vi "REPL_Comm.vi"(8 "REPL Name":string="Robot  REPL", 9 "CodeRef":refnum<vi>, 11 "Microprocessor in":T2) -> (3 "Microprocessor out":T2)   [LabVIEW 2016]
uses:
  uPythonX/uPythonX.xctl
  uPythonX/PythonData.ctl
  <vilib>/event_ctls.llb/eventvkey.ctl
  <vilib>/Utility/miscctls.llb/LVPointTypeDef.ctl
panel:
  in  "Find Port":bool
  out "return?":bool
  in  "Board":bool
  out "mouse down?":bool
  in  "Port":string
  in  "Delete":bool
  in  "New":bool
  in  "Files":u16(ring) items=["Current Code", "LPF2Class.py", "README.txt", "main.py"]
  in  "Ctrls":T1(ring)
  out "rows":string
  in  "View":u16(ring) items=["Complete Code"]
  in  "Spaces":bool
  in  "HelpCode":string
  in  "Stop Script":bool
  in  "Pause":bool
  in  "Help Button":bool
  in  "refresh":bool
  in  "Code":string
  out "Script":string
  in  "Copy":bool
  out "String":string
  in  "Run":bool
  out "FullCode":string
  in  "Clear":bool
  out "Origin":T3
  in  "Ctrl D":bool
  in  "Ctrl C":bool
  in  "Run DIrect":bool
  in  "Main":bool
  out "Console":string
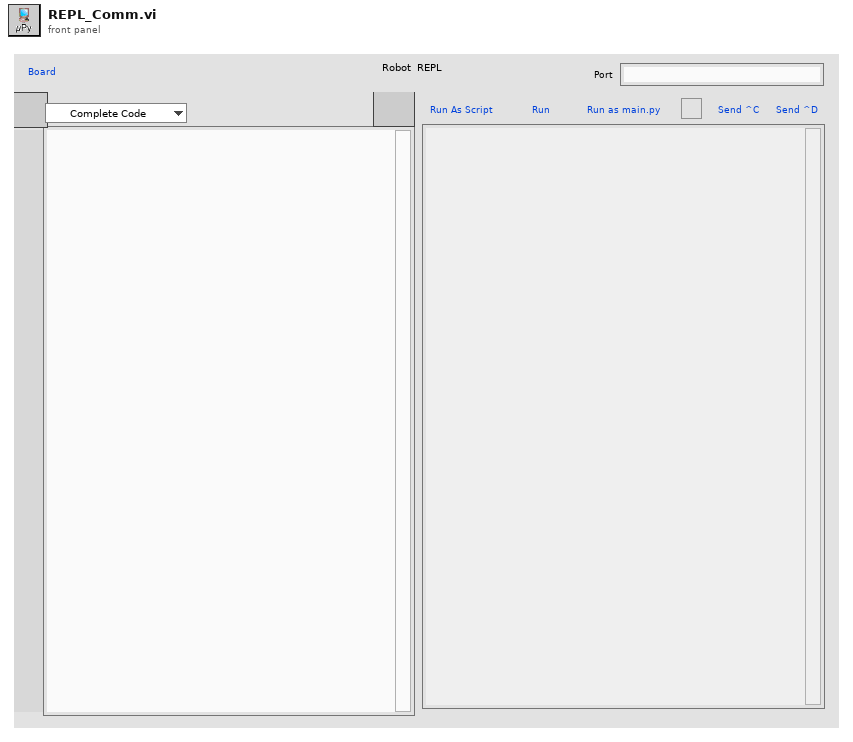
[diagram p1: front panel]
types:
  T1 = enum16{"File Control", "Save to PC", "Read from PC", "Save to MP as..."}
  T2 = cluster{"VISA Refnum in":refnum<visa-resource-name>, "Python Code":string}
  T3 = typedef "LVPointTypeDef.ctl" = cluster{"Horizontal":i16, "Vertical":i16}
  T4 = typedef "uPythonX.xctl/PythonData.ctl" = cluster{"Port":refnum<visa-resource-name>, "All Code":string}
  T5 = typedef "eventvkey.ctl" = enum16{"ASCII", "Enter", "Return", "Shift", "Ctrl", "Alt", "Cmd", "Opt", "Caps", "NumLock", "Clear", "Break", "Up", "Down", "Left", "Right", "Insert", "Delete", "Home", "End", "PageUp", "PageDown", "Escape", "Help", "Pause", "ScrollLock", "F1", "F2", "F3", "F4", "F5", "F6", "F7", "F8", "F9", "F10", "F11", "F12", "F13", "F14", "F15", "F16", "F17", "F18", "F19", "F20", "F21", "F22", "F23", "F24", "Play", "VolumeUp", "VolumeDown", "Mute", "Two Byte Char"}
  T6 = cluster{"Shift":bool, "Ctrl":bool, "Alt":bool, "Cmd":bool, "Opt":bool}
  T7 = cluster{"Char":i16, "VKey":T5, "ScanCode":i16, "Mods":cluster{"Num Pad":bool, "Menu Key":bool}, "PlatMods":cluster{"Shift":bool, "Ctrl":bool, "Alt":bool, "Cmd":bool, "Opt":bool}, "FocusObj":refnum<vi>}
  T8 = enum16{"Left Button", "Center Button", "Right Button", "Window Close"}
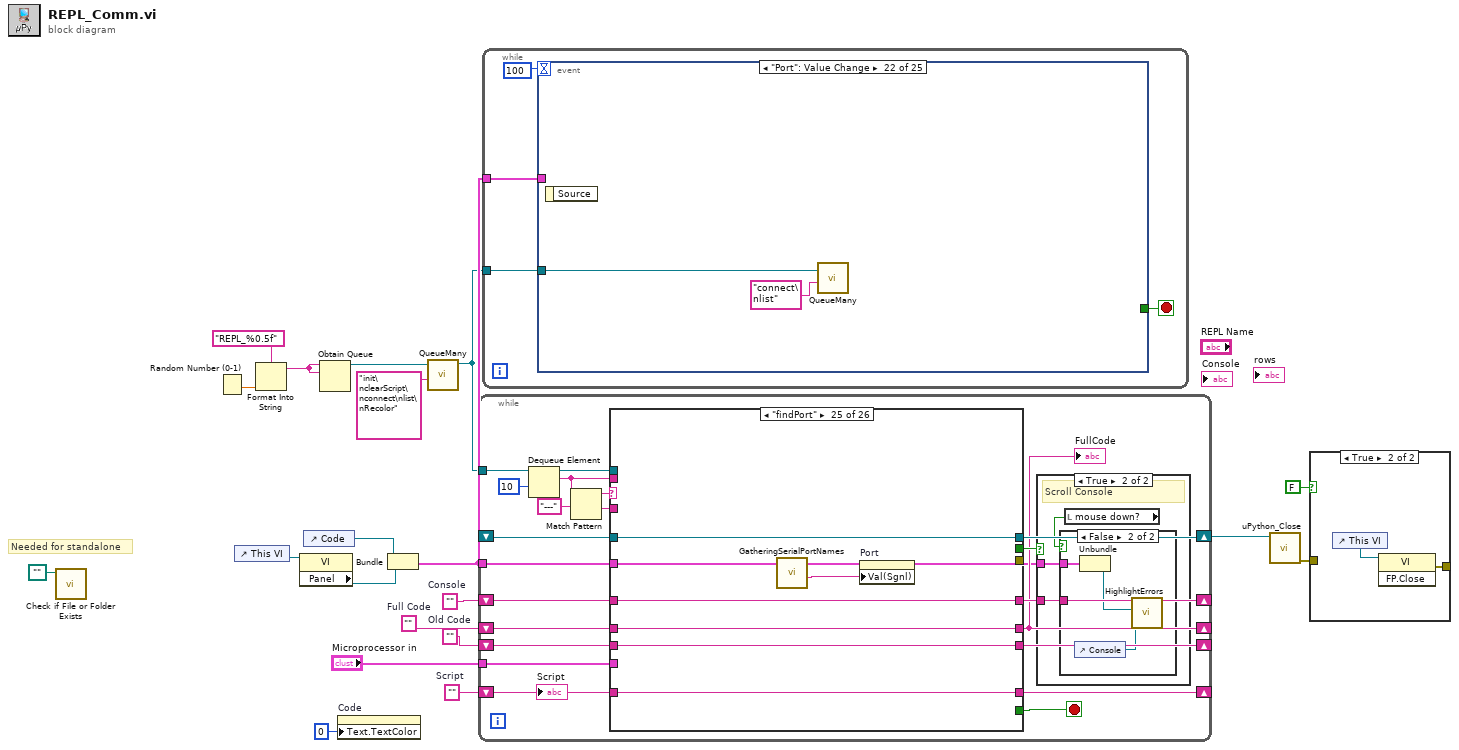
[diagram p0: block diagram]
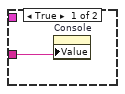
[diagram p4: hidden frame]
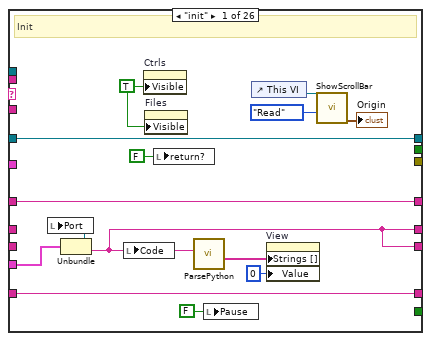
[diagram p5: hidden frame]
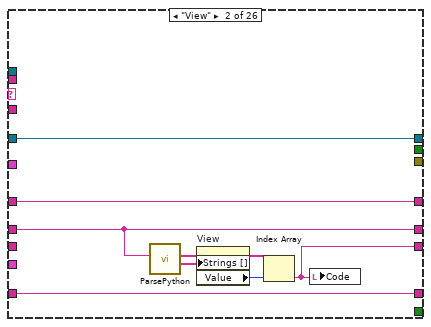
[diagram p6: hidden frame]
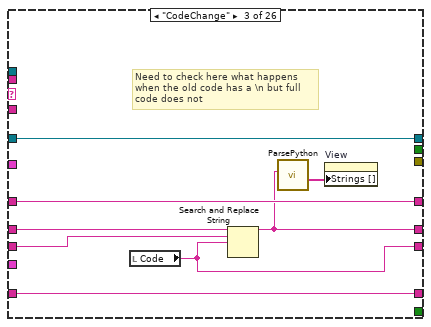
[diagram p7: hidden frame]
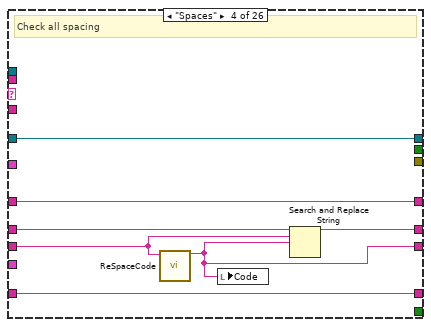
[diagram p8: hidden frame]
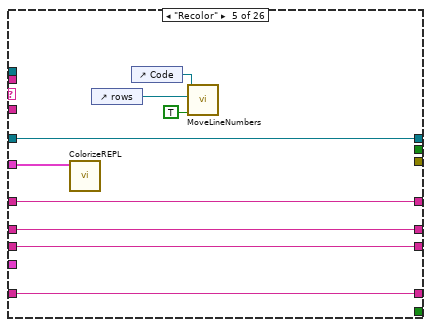
[diagram p9: hidden frame]
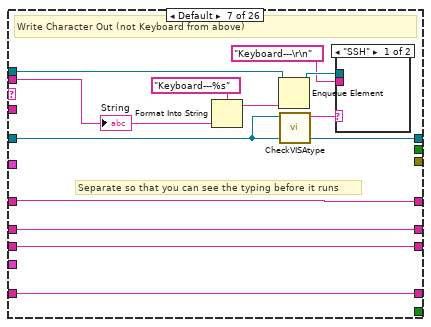
[diagram p11: hidden frame]
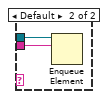
[diagram p12: hidden frame]
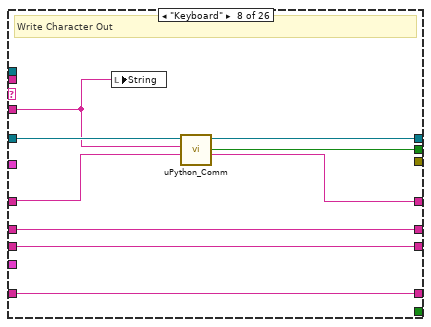
[diagram p13: hidden frame]
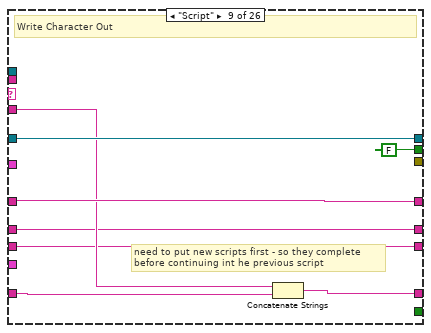
[diagram p14: hidden frame]
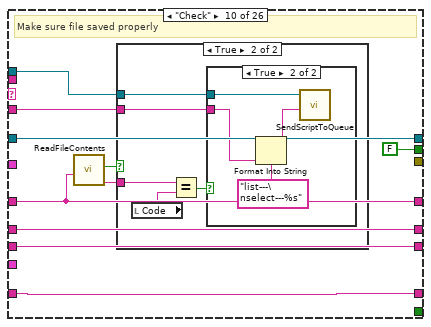
[diagram p15: hidden frame]
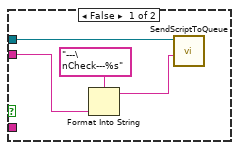
[diagram p16: hidden frame]
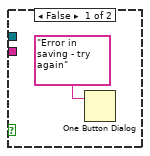
[diagram p17: hidden frame]
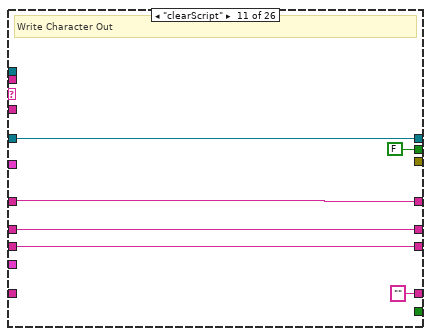
[diagram p18: hidden frame]
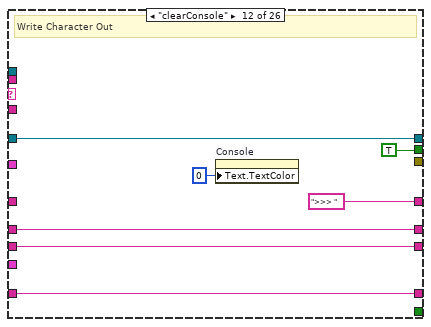
[diagram p19: hidden frame]
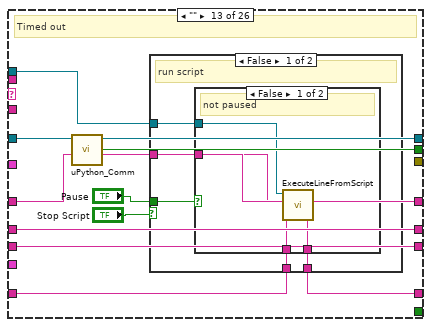
[diagram p20: hidden frame]
diagram:
  w6 = ""  # Old Code
  w7 = ""  # Full Code
  w15 = ""  # Script
  w16 = ""  # Console
  # "Needed for standalone"
  n1 = call <vilib>:"Check if File or Folder Exists.vi"("path"=path "") -> ()  [unwired: 8 in, 3 out]
  n2 = Random Number (0-1)() -> (number: 0 to 1=w10:dbl)
  n3 = control-ref of="This VI"() -> (w5:refnum<vi>)
  n4 = Format Into String(format string="REPL_%0.5f" ("name (unnamed)"), w10) -> (resulting string=w9:string)  [unwired: 2 in, 1 out]
  n5 = property class="VI"(reference=w5) -> ("Panel"=w3:refnum<vi>)  [unwired: 1 in, 2 out]
  n6 = control-ref of="Code"() -> (w4:refnum<vi>)
  n7 = Obtain Queue(name (unnamed)=w9, element data type=w9) -> (queue out=w19:refnum<queue>)  [unwired: 3 in, 2 out]
  n8 = property on="Code" class="Str"("Text.TextColor"=u32 0 ("Text.Text Colors:Text Color")) -> ()  [unwired: 2 in, 2 out]
  n9 = Bundle("Code"=w4, "Panel"=w3) -> (w20:cluster{"Code":refnum<vi>, "Panel":refnum<vi>})  [unwired: 1 in]
  n10 = call "QueueMany.vi"("Playlist"="init\nclearScript\nconnect\nlist\nRecolor" ("element"), "Queue in"=w19) -> ("Queue out"=w18:refnum<queue>)  [unwired: 9 in]
  n11 = while {
    tunnel: w18 -> [w41]
    shift-right: [w31] -> w17
    shift-left: _ -> [w39]
    shift-right: [w30] -> _
    shift-left: w16 -> [w32]
    shift-right: [w28] -> _
    shift-left: w15 -> [w27]
    tunnel: "Microprocessor in" -> [w26]
    shift-right: [w24] -> _
    shift-left: w7 -> [w25]
    shift-right: [w23] -> _
    shift-left: w6 -> [w22]
    tunnel: w20 -> [w21]
    stop <- w40 stop-if-true
    n12 = Dequeue Element(queue=w41, timeout in ms (-1)=10) -> (queue out=w37:refnum<queue>, element=w33:string)  [unwired: 1 in, 2 out]
    n13 = Match Pattern(string=w33, regular expression="---") -> (before substring=w35:string, after substring=w34:string)  [unwired: 1 in, 2 out]
    n14 = case shown="\"findPort\"" w35 {
      tunnel: [_ _ _ _ _ _ _ _ _ _ _ _ _ _ _ _ _ _ _ _ _ _ _ _ _ TRUE] -> w40
      tunnel: w39 -> [w63 w71 w79 w86 w95 w100 w102 w122 w131 w141 w161 w168 w178 _ w207 w221 w236 w244 w248 w276 w289 w300 w310 w316 w322 w336]
      tunnel: w37 -> [_ _ _ _ _ _ w105 _ _ w137 _ _ w169 _ w211 w218 w233 _ _ _ _ _ _ _ _ _]
      tunnel: w34 -> [_ _ _ _ _ _ _ w117 w126 w134 _ _ _ _ _ _ _ _ _ _ _ w301 _ _ _ _]
      tunnel: w33 -> [_ _ _ _ _ _ w107 _ _ _ _ _ _ _ _ _ _ _ _ _ _ _ _ _ _ _]
      tunnel: [w63 w71 w79 w86 w95 w100 w102 w120 w131 w141 w161 w168 w175 w203 w207 w221 w236 w244 w256 w280 w286 w300 w310 w316 w322 w336] -> w31
      tunnel: w32 -> [w62 w70 w78 w85 w94 w99 w111 w121 w130 w136 w160 _ w177 _ w210 w220 w235 w243 w251 w277 w290 w299 w312 w318 w324 w337]
      tunnel: [w62 w70 w78 w85 w94 w99 w111 w119 w130 w136 w160 ">>> " ("Console") w176 w201 w210 w220 w235 w243 w254 w264 w284 w299 w312 w318 w324 w337] -> w30
      tunnel: [_ _ _ _ _ _ _ _ _ _ _ _ _ w202 _ _ _ _ w253 w279 w285 _ _ _ _ _] -> _
      tunnel: [_ _ _ _ _ _ _ w118 FALSE ("Update?") FALSE ("Update?") FALSE ("Update?") TRUE ("Update?") w174 _ TRUE ("Update?") FALSE ("Update?") _ _ TRUE ("Update?") TRUE ("Update?") TRUE ("Update?") _ _ _ _ _] -> w29
      tunnel: [w61 w69 w77 w84 w92 w98 w112 w123 w128 w139 "" ("Script") w166 w180 w200 w212 w222 w237 w240 w262 w282 w292 w298 w311 w317 w323 w334] -> w28
      tunnel: w27 -> [w61 w69 w77 w84 w92 w98 w112 w123 w127 w139 _ w166 w179 w200 w212 w222 w237 w240 w262 w282 w292 w298 w311 w317 w323 w334]
      tunnel: w26 -> [w60 _ _ _ _ _ _ _ _ _ _ _ _ _ _ _ _ _ _ _ _ _ _ _ _ w333]
      tunnel: [w51 w67 w72 w80 w91 w97 w104 w116 w125 w133 w157 w164 w172 w198 w209 w217 w232 w242 w247 w275 w288 w294 w304 w314 w321 w328] -> w24
      tunnel: w25 -> [_ w67 w76 w83 w91 w97 w104 w116 w125 w133 w157 w164 w172 w198 w209 w217 _ w242 w247 w275 w288 w294 w304 w314 w321 w328]
      tunnel: [w51 w64 w74 w81 w93 w96 w103 w115 w124 w132 w156 w163 w171 w197 w208 w216 w232 w241 w246 w274 w287 w293 w303 w313 w320 w327] -> w23
      tunnel: w22 -> [_ _ w75 w82 w93 w96 w103 w115 w124 w132 w156 w163 w171 w197 w208 w216 _ w241 w246 w274 w287 w293 w303 w313 w320 w327]
      tunnel: w21 -> [_ _ _ _ w90 _ _ _ _ _ _ _ _ _ _ _ _ _ _ _ _ _ _ _ _ _]
      frame "init" {
        w58 = TRUE ("Visible")
        # "Init"
        n15 = Unbundle(w60) -> ("VISA Refnum in"=w54:refnum<visa-resource-name>, "Python Code"=w51:string)
        n16 = local write "Port"(w54) -> ()
        n17 = local write "Code"(w51) -> ()
        n18 = property on="Ctrls" class="Enum (strict)"("Visible"=w58) -> ()  [unwired: 2 in, 2 out]
        n19 = property on="Files" class="Ring (strict)"("Visible"=w58) -> ()  [unwired: 2 in, 2 out]
        n20 = local write "return?"(FALSE ("return?")) -> ()
        n21 = call "ParsePython.vi"("String"=w51) -> ("functions"=w53:string[])  [unwired: 8 in, 2 out]
        n22 = local write "Pause"(FALSE ("Pause")) -> ()
        n23 = control-ref of="This VI"() -> (w57:refnum<vi>)
        n24 = property on="View" class="Ring (strict)"("Strings []"=w53, "Value"=0 ("timeout in ms (-1)")) -> ()  [unwired: 2 in, 2 out]
        n25 = call "ShowScrollBar.vi"("Task"=enum16{"Read", "Open", "Close", "Reset"}."Read", "VI in"=w57) -> ("Origin"=→"Origin":T3)  [unwired: 9 in]
      }
      frame "View" {
        n26 = call "ParsePython.vi"("String"=w67) -> ("functions"=w66:string[], "Subs"=w65:string[])  [unwired: 8 in, 1 out]
        n27 = property on="View" class="Ring (strict)"("Strings []"=w66) -> ("Value"=w68:u16)  [unwired: 2 in, 2 out]
        n28 = Index Array(array=w65, index=w68) -> (element=w64:string)
        n29 = local write "Code"(w64) -> ()
      }
      frame "CodeChange" {
        # "Need to check here what happens\nwhen the old code has a \\n but full\ncode does not"
        n30 = local read "Code"() -> (w74:string)
        n31 = Search and Replace String(input string=w76, search string=w75, replace string=w74) -> (result string=w72:string)  [unwired: 5 in, 3 out]
        n32 = call "ParsePython.vi"("String"=w72) -> ("functions"=w73:string[])  [unwired: 8 in, 2 out]
        n33 = property on="View" class="Ring (strict)"("Strings []"=w73) -> ()  [unwired: 2 in, 2 out]
      }
      frame "Spaces" {
        # "Check all spacing"
        n34 = call "ReSpaceCode.vi"("Code"=w82) -> ("String"=w81:string)  [unwired: 10 in]
        n35 = local write "Code"(w81) -> ()
        n36 = Search and Replace String(input string=w83, search string=w82, replace string=w81) -> (result string=w80:string)  [unwired: 5 in, 3 out]
      }
      frame "Recolor" {
        n37 = call "ColorizeREPL.vi"("refs"=w90) -> ()  [unwired: 9 in, 1 out]
        n38 = control-ref of="rows"() -> (w88:refnum<vi>)
        n39 = control-ref of="Code"() -> (w89:refnum<vi>)
        n40 = call "MoveLineNumbers.vi"("Force?"=TRUE, "rows"=w88, "Code"=w89) -> ()  [unwired: 9 in]
      }
      frame "scroll" {
        # "reset row numbers"
      }
      frame Default {
        # "Separate so that you can see the typing before it runs"
        # "Write Character Out (not Keyboard from above)"
        n41 = Format Into String(format string="Keyboard---%s", w107) -> (resulting string=w109:string)  [unwired: 2 in, 1 out]
        n42 = Enqueue Element(queue=w105, element=w109) -> (queue out=w108:refnum<queue>)  [unwired: 2 in, 2 out]
        n43 = call "CheckVISAtype.vi"("VISA Refnum in"=w102) -> ("data string"=w101:string)  [unwired: 9 in, 1 out]
        n44 = case shown="\"SSH\"" w101 {
          tunnel: w108 -> [_ w114]
          tunnel: "Keyboard---\r\n" ("regular expression") -> [_ w113]
          frame "SSH" {
          }
          frame Default {
            n45 = Enqueue Element(queue=w114, element=w113) -> ()  [unwired: 2 in, 3 out]
          }
        }
        "String" <- w107
      }
      frame "Keyboard" {
        # "Write Character Out"
        n46 = local write "String"(w117) -> ()
        n47 = call "uPython_Comm.vi"("Console In"=w121, "Script"=w117, "VISA Refnum in"=w122) -> ("Console Out"=w119:string, "VISA out"=w120:refnum<visa-resource-name>, "Update?"=w118:bool)  [unwired: 4 in, 2 out]
      }
      frame "Script" {
        # "need to put new scripts first - so they complete\nbefore continuing int he previous script"
        # "Write Character Out"
        n48 = Concatenate Strings(w126, w127) -> (w128:string)
      }
      frame "Check" {
        # "Make sure file saved properly"
        n49 = call "ReadFileContents.vi"("Console"=w136) -> ("File Contents"=w135:string, "Success?"=w138:bool)  [unwired: 9 in]
        n50 = case shown="True" w138 {
          tunnel: w137 -> [w145 w146]
          tunnel: w135 -> [_ w149]
          tunnel: w134 -> [w143 w148]
          frame False {
            n51 = Format Into String(format string="---\nCheck---%s" ("String"), w143) -> (resulting string=w142:string)  [unwired: 2 in, 1 out]
            n52 = call "SendScriptToQueue.vi"("String"=w142, "Queue in"=w145) -> ()  [unwired: 10 in]
          }
          frame True {
            n53 = local read "Code"() -> (w150:string)
            n54 = Equal?(x=w149, y=w150) -> (x = y?=w147:bool)
            n55 = case shown="True" w147 {
              tunnel: w148 -> [_ w154]
              tunnel: w146 -> [_ w153]
              frame False {
                n56 = One Button Dialog(message="Error in saving - try again" ("Code")) -> ()  [unwired: 1 in, 1 out]
              }
              frame True {
                n57 = Format Into String(format string="list---\nselect---%s" ("element"), w154) -> (resulting string=w152:string)  [unwired: 2 in, 1 out]
                n58 = call "SendScriptToQueue.vi"("String"=w152, "Queue in"=w153) -> ()  [unwired: 10 in]
              }
            }
          }
        }
      }
      frame "clearScript" {
        # "Write Character Out"
      }
      frame "clearConsole" {
        # "Write Character Out"
        n59 = property on="Console" class="Str"("Text.TextColor"=u32 0 ("Text.Text Colors:Text Color")) -> ()  [unwired: 2 in, 2 out]
      }
      frame "" {
        # "Timed out"
        n60 = call "uPython_Comm.vi"("Console In"=w177, "VISA Refnum in"=w178) -> ("Console Out"=w176:string, "VISA out"=w175:refnum<visa-resource-name>, "Update?"=w174:bool)  [unwired: 5 in, 2 out]
        n61 = case shown="False" "Stop Script" {
          tunnel: [w185 "" ("Script")] -> w180
          tunnel: w179 -> [w184 _]
          tunnel: w176 -> [w183 _]
          tunnel: "Pause" -> [w182 _]
          tunnel: w169 -> [w181 _]
          frame False {
            # "run script"
            n62 = case shown="False" w182 {
              tunnel: [w189 w190] -> w185
              tunnel: w184 -> [w188 w190]
              tunnel: w183 -> [w187 _]
              tunnel: w181 -> [w186 _]
              frame False {
                # "not paused"
                n63 = call "ExecuteLineFromScript.vi"("Script in"=w188, "Console"=w187, "Queue in"=w186) -> ("Script out"=w189:string)  [unwired: 8 in]
              }
              frame True {
              }
            }
          }
          frame True {
          }
        }
      }
      frame "connect" {
        w201 = "" ("element")
        n64 = property on="Files" class="Ring (strict)"("Strings []"=string[] [] ("Item Names")) -> ()  [unwired: 2 in, 2 out]
        n65 = Match Pattern(string="Port", regular expression="- ") -> (after substring=w192:string, offset past match=w195:i32)  [unwired: 1 in, 2 out]
        n66 = case shown="0, Default" w195 {
          tunnel: "Port" -> [_ w205]
          tunnel: [w204 w205] -> w193
          tunnel: w192 -> [w204 _]
          frame 0, Default {
          }
          frame -1 {
          }
        }
        n67 = local write "Console"(w201) -> ()
        n68 = call "uPython_Initialize.vi"("VISA Refnum in"=w193) -> ("error out"=w202:errorcluster, "VISA Refnum out"=w203:refnum<visa-resource-name>)  [unwired: 9 in]
      }
      frame "list" {
        # "get file listing"
        n69 = call "CheckVISAtype.vi"("VISA Refnum in"=w207) -> ("data string"=w206:string)  [unwired: 9 in, 1 out]
        n70 = case shown="Default" w206 {
          tunnel: w211 -> [w215 _]
          frame Default {
            n71 = call "SendScriptToQueue.vi"("String"="import os\nos.listdir()\n\nlisting---" ("element"), "Queue in"=w215) -> ()  [unwired: 10 in]
          }
          frame "" {
          }
        }
      }
      frame "listing" {
        # "get file listing"
        n72 = call "GetFileListing.vi"("Console In"=w220) -> ("Files"=w224:string[], "Success?"=w219:bool)  [unwired: 9 in]
        n73 = case shown="True" w219 {
          tunnel: w224 -> [_ w230]
          tunnel: w218 -> [w225 _]
          frame False {
            n74 = call "SendScriptToQueue.vi"("String"="---\nlisting---", "Queue in"=w225) -> ()  [unwired: 10 in]
          }
          frame True {
            n75 = Build Array (concatenate)("Current Code", w230) -> (w229:string[])
            n76 = property on="Files" class="Ring (strict)"("Strings []"=w229, "Val(Sgnl)"=0) -> ()  [unwired: 2 in, 2 out]
          }
        }
      }
      frame "read" {
        n77 = call "ReadFileContents.vi"("Console"=w235) -> ("File Contents"=w232:string, "Success?"=w234:bool)  [unwired: 9 in]
        n78 = local write "Code"(w232) -> ()
        n79 = case shown="False" w234 {
          tunnel: w233 -> [w239 _]
          frame False {
            n80 = call "SendScriptToQueue.vi"("String"="---\nread---", "Queue in"=w239) -> ()  [unwired: 10 in]
          }
          frame True {
          }
        }
        n81 = property on="View" class="Ring (strict)"("Val(Sgnl)"=0 ("timeout in ms (-1)")) -> ()  [unwired: 2 in, 2 out]
      }
      frame "ListDialog" {
        n82 = call "ReadFilesOnMP.vi"("VISA"=w244) -> ()  [unwired: 11 in]
      }
      frame "run" {
        w252 = "\u0003"  # Ctrl C
        w259 = "\u0004"  # Ctrl D
        # "run on main.py"
        n83 = call "uPython_Comm.vi"("Console In"=w251, "Script"=w252, "VISA Refnum in"=w248) -> ("error out"=w250:errorcluster, "VISA out"=w249:refnum<visa-resource-name>)  [unwired: 4 in, 3 out]
        n84 = local read "Code"() -> (w255:string)
        n85 = call "SavePyFile.vi"("Name"="main.py", "error in"=w250, "Python Code"=w255, "VISA in"=w249) -> ("error out"=w260:errorcluster, "Reply"=w258:string, "VISA out"=w261:refnum<visa-resource-name>)  [unwired: 5 in]
        n86 = call "uPython_Comm.vi"("error in (no error)"=w260, "Console In"=w258, "Script"=w259, "VISA Refnum in"=w261) -> ("error out"=w253:errorcluster, "Console Out"=w254:string, "VISA out"=w256:refnum<visa-resource-name>)  [unwired: 3 in, 2 out]
      }
      frame "runRaw" {
        w278 = "\u0003\u0003\u0001"  # Ctrl C,C,A
        w281 = "\u0004"  # Ctrl D
        # "run on main.py"
        n87 = call "uPython_Comm.vi"("Console In"=w277, "Script"=w278, "VISA Refnum in"=w276) -> ("error out"=w272:errorcluster, "Console Out"=w268:string, "VISA out"=w273:refnum<visa-resource-name>)  [unwired: 4 in, 2 out]
        n88 = local read "Code"() -> (w269:string)
        n89 = call "uPython_Comm.vi"("error in (no error)"=w272, "Console In"=w268, "Script"=w269, "VISA Refnum in"=w273) -> ("error out"=w271:errorcluster, "Console Out"=w267:string, "VISA out"=w270:refnum<visa-resource-name>)  [unwired: 3 in, 2 out]
        n90 = call "uPython_Comm.vi"("error in (no error)"=w271, "Console In"=w267, "Script"=w281, "VISA Refnum in"=w270) -> ("error out"=w279:errorcluster, "Console Out"=w265:string, "VISA out"=w280:refnum<visa-resource-name>)  [unwired: 3 in, 2 out]
        n91 = Concatenate Strings(w265, "\r\n" ("Script")) -> (w264:string)
      }
      frame "leaveRaw" {
        w291 = "\r\u0002"  # \r Ctrl B
        # "run on main.py"
        n92 = call "uPython_Comm.vi"("Console In"=w290, "Script"=w291, "VISA Refnum in"=w289) -> ("error out"=w285:errorcluster, "Console Out"=w284:string, "VISA out"=w286:refnum<visa-resource-name>)  [unwired: 4 in, 2 out]
      }
      frame "select" {
        n93 = property on="Files" class="Ring (strict)"() -> ("Strings []"=w295:string[])  [unwired: 2 in, 2 out]
        n94 = call <vilib>:"Trim Whitespace.vi"("string"=w301) -> ("trimmed string"=w297:string)  [unwired: 1 in]
        n95 = Search 1D Array(1D array=w295, element=w297) -> (index of element=w296:i32)  [unwired: 1 in]
        n96 = case shown="Default" w296 {
          selector: w296 -> [_ w302]
          frame -1 {
          }
          frame Default {
            n97 = property on="Files" class="Ring (strict)"("Val(Sgnl)"=w302) -> ()  [unwired: 2 in, 2 out]
          }
        }
      }
      frame "help" {
        n98 = local read "Code"() -> (w305:string)
        n99 = Bundle(cluster=T4 {"Port"="", "All Code"="Hi"} ("Data In"), "Port"=w310, "All Code"=w305) -> (w309:T4)
        n100 = control-ref of="HelpCode"() -> (w307:refnum<vi>)
        n101 = call "OpenHelp.vi"("Code Ref"=w307, "Data In"=w309, "Dialog"=enum16{"REPL", "Help"}."Help") -> ()  [unwired: 9 in]
      }
      frame "update" {
        n102 = property class="Str"(reference="CodeRef", "Val(Sgnl)"=w314) -> ()  [unwired: 1 in, 2 out]
      }
      frame "findPort" {
        n103 = call "GatheringSerialPortNames.vi"() -> ("name"=w319:string)  [unwired: 11 in]
        n104 = property on="Port" class="Str"("Val(Sgnl)"=w319) -> ()  [unwired: 2 in, 2 out]
      }
      frame "done" {
        w332 = FALSE ("Visible")
        n105 = property on="Code" class="Str"("Value"="" ("Code"), "Text.TextColor"=u32 0 ("Text.Text Colors:Text Color")) -> ()  [unwired: 2 in, 2 out]
        n106 = property on="Ctrls" class="Enum (strict)"("Visible"=w332) -> ()  [unwired: 2 in, 2 out]
        n107 = Bundle(cluster=w333, "VISA Refnum in"=w336, "Python Code"=w328) -> (→"Microprocessor out":T2)
        n108 = property on="Files" class="Ring (strict)"("Visible"=w332) -> ()  [unwired: 2 in, 2 out]
        n109 = control-ref of="This VI"() -> (w330:refnum<vi>)
        n110 = local read "Origin"() -> (w331:T3)
        n111 = call "ShowScrollBar.vi"("Origin in"=w331, "Task"=enum16{"Read", "Open", "Close", "Reset"}."Reset", "VI in"=w330) -> ()  [unwired: 8 in, 1 out]
      }
    }
    "FullCode" <- w24
    n112 = case shown="True" w29 {
      tunnel: w30 -> [_ w44]
      tunnel: w21 -> [_ w42]
      frame False {
      }
      frame True {
        # "Scroll Console"
        n113 = local read "mouse down?"() -> (w43:bool)
        n114 = case shown="False" w43 {
          tunnel: w44 -> [w45 w49]
          tunnel: w42 -> [_ w47]
          frame True {
            n115 = property on="Console" class="Str"("Value"=w45) -> ()  [unwired: 2 in, 2 out]
          }
          frame False {
            n116 = control-ref of="Console"() -> (w48:refnum<vi>)
            n117 = Unbundle(w47) -> ("Panel"=w46:refnum<vi>)  [unwired: 1 out]
            n118 = call "HighlightErrors.vi"("String"=w49, "Front Panel"=w46, "Console"=w48) -> ()  [unwired: 9 in]
          }
        }
      }
    }
    "Script" <- w27
  }
  n119 = while {
    tunnel: w18 -> [w342]
    tunnel: w20 -> [w339]
    stop <- w341 stop-if-true
    n120 = event shown="[21] \"Port\": Value Change" {
      selector: _ -> [_ _ _ _ _ _ _ _ _ _ _ _ _ _ _ _ _ _ _ _ _ _ _ _ _]
      dyn-events: _ -> [_ _ _ _ _ _ _ _ _ _ _ _ _ _ _ _ _ _ _ _ _ _ _ _ _]
      timeout: 100 -> [_ _ _ _ _ _ _ _ _ _ _ _ _ _ _ _ _ _ _ _ _ _ _ _ _]
      tunnel: w342 -> [_ w348 w351 w353 w359 w388 _ _ w398 w414 w420 w422 w424 w428 w452 w456 w458 w459 w461 w468 w475 w476 w478 _ w481]
      tunnel: [_ _ _ _ _ _ _ _ w391 _ _ _ _ _ _ _ _ _ _ _ _ _ _ _ _] -> w341
      tunnel: w339 -> [_ w347 _ _ _ _ _ _ _ _ _ _ _ _ _ _ _ _ _ _ _ _ _ _ _]
      event Timeout {
        n121 = event-data() -> ()  [unwired: 1 in, 3 out]
        n122 = control-ref of="Code"() -> (w344:refnum<vi>)
        n123 = control-ref of="rows"() -> (w345:refnum<vi>)
        n124 = call "MoveLineNumbers.vi"("Force?"=TRUE, "rows"=w345, "Code"=w344) -> ()  [unwired: 9 in]
      }
      event "Code": Value Change {
        # "Need to have these here or you can get screwy stuff happening"
        n125 = event-data() -> ()  [unwired: 1 in, 2 out]
        n126 = local read "return?"() -> (w346:bool)
        n127 = call "ColorizeREPL.vi"("refs"=w347, "Add Spaces?"=w346) -> ()  [unwired: 8 in, 1 out]
        n128 = call "QueueMany.vi"("Playlist"="CodeChange" ("element"), "Queue in"=w348) -> ()  [unwired: 9 in, 1 out]
      }
      event "View": Value Change {
        n129 = event-data() -> ()  [unwired: 1 in, 1 out]
        n130 = call "QueueMany.vi"("Playlist"="View\nRecolor" ("element"), "Queue in"=w351) -> ()  [unwired: 9 in, 1 out]
      }
      event "Spaces": Value Change {
        n131 = event-data() -> ()  [unwired: 1 in, 1 out]
        n132 = call "QueueMany.vi"("Playlist"="Spaces\nRecolor" ("element"), "Queue in"=w353) -> ()  [unwired: 9 in, 1 out]
      }
      event Key Down {
        n133 = event-data() -> ("Char"=w363:i16, "VKey"=w355:T5, "ScanCode"=w362:i16, "Mods"=w361:cluster{"Num Pad":bool, "Menu Key":bool}, "PlatMods"=w360:T6, "FocusObj"=w356:refnum<vi>)  [unwired: 1 in]
        n134 = case shown="\"F4\"" w355 {
          frame "ASCII", Default {
          }
          frame "F4" {
            n135 = control-ref of="This VI"() -> (w366:refnum<vi>)
            n136 = property on="Ctrls" class="Enum (strict)"() -> ("Visible"=w367:bool)  [unwired: 2 in, 2 out]
            n137 = case shown="False" w367 {
              tunnel: [FALSE ("Visible") TRUE ("Visible")] -> w365
              tunnel: w366 -> [w370 w374]
              frame True {
                n138 = local read "Origin"() -> (w369:T3)
                n139 = call "ShowScrollBar.vi"("Origin in"=w369, "Task"=enum16{"Read", "Open", "Close", "Reset"}."Close", "VI in"=w370) -> ()  [unwired: 8 in, 1 out]
              }
              frame False {
                n140 = local read "Origin"() -> (w373:T3)
                n141 = call "ShowScrollBar.vi"("Origin in"=w373, "Task"=enum16{"Read", "Open", "Close", "Reset"}."Open", "VI in"=w374) -> ()  [unwired: 8 in, 1 out]
              }
            }
            n142 = property on="Ctrls" class="Enum (strict)"("Visible"=w365) -> ()  [unwired: 2 in, 2 out]
            n143 = property on="Files" class="Ring (strict)"("Visible"=w365) -> ()  [unwired: 2 in, 2 out]
          }
        }
        n144 = Bundle("Char"=w363, "VKey"=w355, "ScanCode"=w362, "Mods"=w361, "PlatMods"=w360, "FocusObj"=w356) -> (w364:T7)  [unwired: 1 in]
        n145 = control-ref of="Code"() -> (w357:refnum<vi>)
        n146 = Not Equal?(x=w357, y=w356) -> (x != y?=w358:bool)
        n147 = case shown="True" w358 {
          tunnel: w364 -> [_ w382]
          tunnel: w359 -> [_ w380]
          tunnel: w355 -> [w377 _]
          tunnel: [w376 _] -> w354
          frame False {
            n148 = Equal?(x=eventvkey."Return" ("VKey"), y=w377) -> (x = y?=w376:bool)
          }
          frame True {
            n149 = call "TranslateTyping.vi"("Cluster"=w382) -> ("Script?"=w379:bool, "string"=w381:string)  [unwired: 8 in, 1 out]
            n150 = case shown="True" w379 {
              tunnel: w381 -> [w383 w386]
              tunnel: w380 -> [w384 w385]
              frame False {
                n151 = call "QueueMany.vi"("Playlist"=w383, "Queue in"=w384) -> ()  [unwired: 9 in, 1 out]
              }
              frame True {
                n152 = call "SendScriptToQueue.vi"("String"=w386, "Queue in"=w385) -> ()  [unwired: 10 in]
              }
            }
          }
        }
        "return?" <- w354
      }
      event "Copy": Value Change {
        n153 = event-data() -> ()  [unwired: 1 in, 1 out]
        n154 = call "QueueMany.vi"("Playlist"="update" ("element"), "Queue in"=w388) -> ()  [unwired: 9 in, 1 out]
      }
      event Mouse Down {
        n155 = event-data() -> ()  [unwired: 1 in, 8 out]
        "mouse down?" <- TRUE ("mouse down?")
      }
      event Mouse Leave; Mouse Up {
        n156 = event-data() -> ()  [unwired: 1 in, 4 out]
        n157 = local write "mouse down?"(FALSE ("mouse down?")) -> ()
      }
      event Panel Close? {
        n158 = event-data() -> ()  [unwired: 1 in, 1 out]
        n159 = local read "Microprocessor in"() -> (w395:T2)
        n160 = local read "Code"() -> (w394:string)
        n161 = Unbundle By Name(w395) -> ("Python Code"=w393:string)
        n162 = Not Equal?(x=w393, y=w394) -> (x != y?=w392:bool)
        n163 = case shown="True" w392 {
          tunnel: ["done" ("element") w403] -> w396
          tunnel: [TRUE ("Discard?") w402] -> w391
          frame False {
          }
          frame True {
            n164 = call "CloseDialog.vi"() -> ("Which Button?"=w401:T8)  [unwired: 11 in]
            n165 = case shown="\"Center Button\"" w401 {
              tunnel: ["update\ndone" ("element") "done" ("element") "" ("element")] -> w403
              tunnel: [TRUE ("Discard?") TRUE ("Discard?") FALSE ("Discard?")] -> w402
              frame "Left Button" {
              }
              frame "Center Button" {
              }
              frame Default {
              }
            }
          }
        }
        n166 = call "QueueMany.vi"("Playlist"=w396, "Queue in"=w398) -> ()  [unwired: 9 in, 1 out]
        n167 = event-data("Discard?"=TRUE) -> ()  [unwired: 1 in, 1 out]
      }
      event "Files": Value Change {
        n168 = event-data() -> ("OldVal"=w410:u16)  [unwired: 1 in]
        n169 = property on="Files" class="Ring (strict)"() -> ("Strings []"=w412:string[])  [unwired: 2 in, 2 out]
        n170 = Index Array(array=w412, index="Files") -> (element=w411:string)
        n171 = case shown="Default" w411 {
          selector: w411 -> [_ w415]
          tunnel: w414 -> [_ w417]
          tunnel: w410 -> [_ _]
          frame "Current Code" {
          }
          frame Default {
            n172 = Format Into String(format string="Script---file = open('%s','rb')\ntext = file.read()\nfile.close()\n\ntext\nread---" ("write buffer"), w415) -> (resulting string=w416:string)  [unwired: 2 in, 1 out]
            n173 = call "SendScriptToQueue.vi"("String"=w416, "Queue in"=w417) -> ()  [unwired: 10 in]
          }
        }
      }
      event "refresh": Value Change {
        n174 = event-data() -> ()  [unwired: 1 in, 1 out]
        n175 = call "QueueMany.vi"("Playlist"="list" ("element"), "Queue in"=w420) -> ()  [unwired: 9 in, 1 out]
      }
      event "Board": Value Change {
        n176 = event-data() -> ()  [unwired: 1 in, 1 out]
        n177 = call "QueueMany.vi"("Playlist"="ListDialog" ("element"), "Queue in"=w422) -> ()  [unwired: 9 in, 1 out]
      }
      event "Find Port": Value Change {
        n178 = event-data() -> ()  [unwired: 1 in, 1 out]
        n179 = call "QueueMany.vi"("Playlist"="findPort" ("element"), "Queue in"=w424) -> ()  [unwired: 9 in, 1 out]
      }
      event "Ctrls": Value Change {
        n180 = event-data() -> ()  [unwired: 1 in, 1 out]
        n181 = case shown="\"Save to PC\"" "Ctrls" {
          tunnel: w428 -> [_ _ w439 _]
          tunnel: [w429 w430 w438 w441] -> w426
          tunnel: T1."File Control" ("Ctrls") -> [w429 w430 w438 w441]
          frame Default {
            # "Default"
          }
          frame "Read from PC" {
            # "Open PC file"
            n182 = call "File Dialog"("prompt"="Find File") -> ("selected path"=w434:path, "cancelled"=w433:bool, "error out"=w431:errorcluster)  [unwired: 11 in, 1 out]
            n183 = case shown="False" w433 {
              tunnel: w434 -> [w437 _]
              tunnel: w431 -> [_ _]
              frame False {
                n184 = Read from Text File(file (use dialog)=w437, count=-1) -> (text=w436:string)  [unwired: 2 in, 3 out]
                n185 = local write "Code"(w436) -> ()
              }
              frame True {
              }
            }
          }
          frame "Save to MP as..." {
            # "Save As... on MP"
            n186 = local read "Code"() -> (w440:string)
            n187 = call "SaveOnMP.vi"("Contents"=w440, "Queue in"=w439) -> ()  [unwired: 10 in]
          }
          frame "Save to PC" {
            # "Save to PC"
            n188 = call "File Dialog2"("prompt"="Select File") -> ("selected path"=w445:path, "cancelled"=w444:bool, "error out"=w442:errorcluster)  [unwired: 11 in, 1 out]
            n189 = case shown="False" w444 {
              tunnel: w445 -> [w447 _]
              tunnel: w442 -> [_ _]
              frame False {
                n190 = call "AddPyExtension.vi"("selected path"=w447) -> ("dup file"=w446:path)  [unwired: 10 in]
                n191 = local read "Code"() -> (w448:string)
                n192 = Write to Text File(file (use dialog)=w446, text=w448) -> ()  [unwired: 2 in, 3 out]
              }
              frame True {
              }
            }
          }
        }
        n193 = local write "Ctrls"(w426) -> ()
      }
      event "Ctrl C": Value Change {
        w451 = "\u0003"  # Ctrl C
        n194 = event-data() -> ()  [unwired: 1 in, 1 out]
        n195 = call "QueueMany.vi"("Playlist"=w451, "Queue in"=w452) -> ("Queue out"=w450:refnum<queue>)  [unwired: 9 in]
        n196 = call "QueueMany.vi"("Playlist"="clearScript" ("element"), "Queue in"=w450) -> ()  [unwired: 9 in, 1 out]
      }
      event "Ctrl D": Value Change {
        w455 = "\u0004"  # Ctrl D
        n197 = event-data() -> ()  [unwired: 1 in, 1 out]
        n198 = call "QueueMany.vi"("Playlist"=w455, "Queue in"=w456) -> ("Queue out"=w453:refnum<queue>)  [unwired: 9 in]
        n199 = call "QueueMany.vi"("Playlist"="clearScript" ("element"), "Queue in"=w453) -> ()  [unwired: 9 in, 1 out]
      }
      event "Run DIrect": Value Change {
        n200 = event-data() -> ()  [unwired: 1 in, 1 out]
        n201 = call "SendScriptToQueue.vi"("String"="Code", "Queue in"=w458) -> ()  [unwired: 10 in]
      }
      event "Main": Value Change {
        n202 = event-data() -> ()  [unwired: 1 in, 1 out]
        n203 = call "QueueMany.vi"("Playlist"="run" ("element"), "Queue in"=w459) -> ()  [unwired: 9 in, 1 out]
      }
      event "Run": Value Change {
        n204 = event-data() -> ()  [unwired: 1 in, 1 out]
        n205 = call "QueueMany.vi"("Playlist"="runRaw" ("element"), "Queue in"=w461) -> ()  [unwired: 9 in, 1 out]
      }
      event "Delete": Value Change {
        n206 = event-data() -> ()  [unwired: 1 in, 1 out]
        n207 = property on="Files" class="Ring (strict)"() -> ("Strings []"=w464:string[], "Value"=w463:u16)  [unwired: 2 in, 2 out]
        n208 = Index Array(array=w464, index=w463) -> (element=w467:string)
        n209 = Format Into String(format string="Delete %s?", w467) -> (resulting string=w471:string)  [unwired: 2 in, 1 out]
        n210 = Format Into String(format string="os.remove('%s')\n\nlist---" ("element"), w467) -> (resulting string=w466:string)  [unwired: 2 in, 1 out]
        n211 = Two Button Dialog(message=w471) -> (T button?=w469:bool)  [unwired: 2 in]
        n212 = case shown="True" w469 {
          tunnel: w468 -> [_ w473]
          tunnel: w466 -> [_ w472]
          frame False {
          }
          frame True {
            n213 = call "SendScriptToQueue.vi"("String"=w472, "Queue in"=w473) -> ()  [unwired: 10 in]
          }
        }
      }
      event "New": Value Change {
        w474 = "# place code here" ("Contents")
        n214 = event-data() -> ()  [unwired: 1 in, 1 out]
        n215 = local write "Code"(w474) -> ()
        n216 = call "SaveOnMP.vi"("Contents"=w474, "Queue in"=w475) -> ()  [unwired: 10 in]
      }
      event "Port": Value Change {
        n217 = event-data() -> ()  [unwired: 1 in, 1 out]
        n218 = call "QueueMany.vi"("Playlist"="connect\nlist" ("element"), "Queue in"=w476) -> ()  [unwired: 9 in, 1 out]
      }
      event "Help Button": Value Change {
        n219 = event-data() -> ()  [unwired: 1 in, 1 out]
        n220 = call "QueueMany.vi"("Playlist"="help" ("element"), "Queue in"=w478) -> ()  [unwired: 9 in, 1 out]
      }
      event "HelpCode": Value Change {
        n221 = event-data() -> ()  [unwired: 1 in, 1 out]
        n222 = property on="Code" class="Str"("Val(Sgnl)"="HelpCode") -> ()  [unwired: 2 in, 2 out]
      }
      event "Clear": Value Change {
        n223 = event-data() -> ()  [unwired: 1 in, 2 out]
        n224 = call "QueueMany.vi"("Playlist"="clearConsole" ("element"), "Queue in"=w481) -> ()  [unwired: 9 in, 1 out]
      }
    }
  }
  n225 = call "uPython_Close.vi"("VISA  in"=w17) -> ("error out"=w13:errorcluster)  [unwired: 9 in, 1 out]
  n226 = case shown="True" FALSE {
    tunnel: w13 -> [_ _]
    tunnel: [_ w483] -> _
    frame False {
    }
    frame True {
      n227 = control-ref of="This VI"() -> (w484:refnum<vi>)
      n228 = invoke class="VI" method="FP.Close"(reference=w484) -> (error out=w483:errorcluster)  [unwired: 2 in, 2 out]
    }
  }
